vi "Robot Global Data.vi"() -> ()   [LabVIEW 2012]
doc: "This global VI can contain as many global variables as you need. Place a control on the panel, give it a good name. To read or write to it from a VI, drag the icon to the diagram of that VI. You can also drag from the project. Click on the node to change which global you access. You shouldn't have multiple locations writing to a global or it will cause a race-condition."
uses:
  <vilib>/Rock Robotics/WPI/Camera/WPI_CameraImageSize.ctl
panel:
  in  "Kinect Array":dbl[](array[numeric])
  out "Kinect Command":string
  in  "Number of Auton Files":i64
  in  "Auton Files":string[](array[string])
  in  "Current File":string
  in  "Auton Array":dbl[][](array[numeric]) format="%0.3f"
  in  "LED toggle rate (ms)":u32=20
  in  "image size":T1=enum."320x240"
  in  "Enable Vision":bool
  # "Z Wrist Right\nZ Wrist Left\nArm (Forward)\nArm (Reverse)"
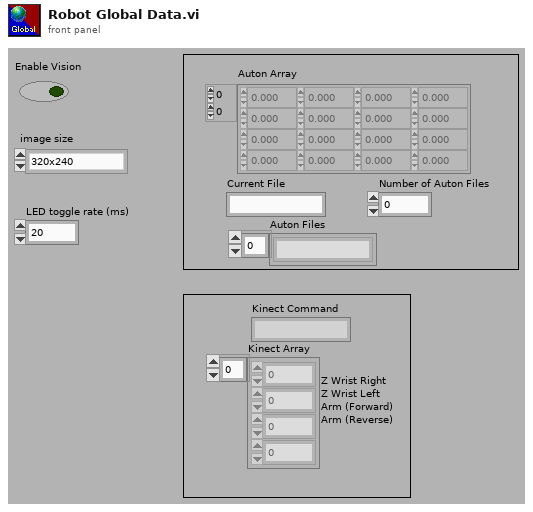
[diagram p1: front panel]
types:
  T1 = typedef "WPI_CameraImageSize.ctl" = enum16{"640x480", "320x240", "160x120"}
diagram:
